vi "Get Parent of Subaddress.vi"(8 "error in":errorcluster, 11 "subaddress":T1 format="%.0x") -> (0 "error out":errorcluster, 2 "parent of subaddress":T1 format="%.0x", 3 "subaddress out":T1 format="%.0x")   [LabVIEW 2020, in "AIM MIL-STD-1553 Scripting.lvlib"]
doc: "Returns the <b>endpoint</b> (terminal address and subaddress) for the parent remote terminal of the <b>subaddress</b>."
uses:
  AIM MIL-STD-1553 Scripting.lvlib
  <vilib>/NI VeriStand/Custom Device API/Custom Device Item Ref.ctl
  Constants.vi
  <vilib>/NI VeriStand/Custom Device API/Custom Device API.lvlib
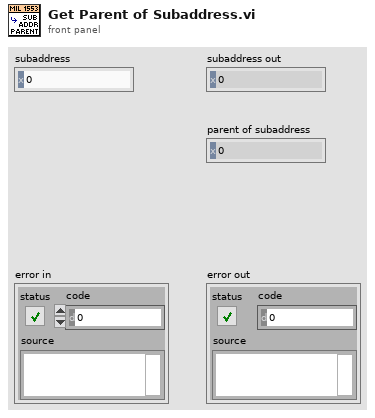
[diagram p1: front panel]
types:
  T1 = typedef "Custom Device API.lvlib/Custom Device Item Ref.ctl" = u64
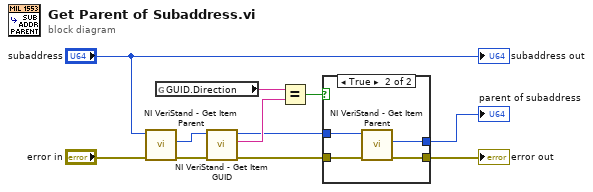
[diagram p0: block diagram]
diagram:
  n1 = call <vilib>:"NI VeriStand - Get Item Parent.vi"("error in (no error)"="error in", "Item Ref in"="subaddress") -> ("error out"=w8:errorcluster, "Parent Ref"=w9:T1)  [unwired: 6 in, 2 out]
  n2 = global read "Constants.vi" "GUID.Direction"() -> (w6:string)
  n3 = call <vilib>:"NI VeriStand - Get Item GUID.vi"("error in (no error)"=w8, "Item Ref in"=w9) -> ("error out"=w3:errorcluster, "GUID"=w7:string, "Item Ref out"=w4:T1)  [unwired: 7 in]
  n4 = Equal?(x=w6, y=w7) -> (x = y?=w5:bool)
  n5 = case shown="True" w5 {
    tunnel: w4 -> [w12 w17]
    tunnel: w3 -> [w13 w16]
    tunnel: [w13 w15] -> w2
    tunnel: [w12 w14] -> w1
    frame False {
    }
    frame True {
      n6 = call <vilib>:"NI VeriStand - Get Item Parent.vi"("error in (no error)"=w16, "Item Ref in"=w17) -> ("error out"=w15:errorcluster, "Parent Ref"=w14:T1)  [unwired: 6 in, 2 out]
    }
  }
  "error out" <- w2
  "parent of subaddress" <- w1
  "subaddress out" <- "subaddress"
